vi "Convert to Lockin Data.vi"(7 "Raw data Y":i32[](array[numeric]), 8 "error in (no error)":errorcluster, 9 "Raw data X":i32[](array[numeric]), 10 "Raw data(F)":i32[](array[numeric]), 11 "RP Transceiver in":refnum<class "RP Transceiver.lvclass">) -> (0 "error out":errorcluster, 1 "Volatge X out":dbl[](array[numeric]), 2 "Frequency out":dbl[](array[numeric]), 3 "RP Transceiver out":refnum<class "RP Transceiver.lvclass">, 4 "Starting edges":i32[](array[numeric]), 5 "Ending edges":i32[](array[numeric]), 6 "Volatge Y out":dbl[](array[numeric]))   [LabVIEW 2024, in "RP Transceiver.lvclass"]
uses:
  RP Transceiver.lvclass
  RP Transceiver.lvclass/RP Transceiver.ctl
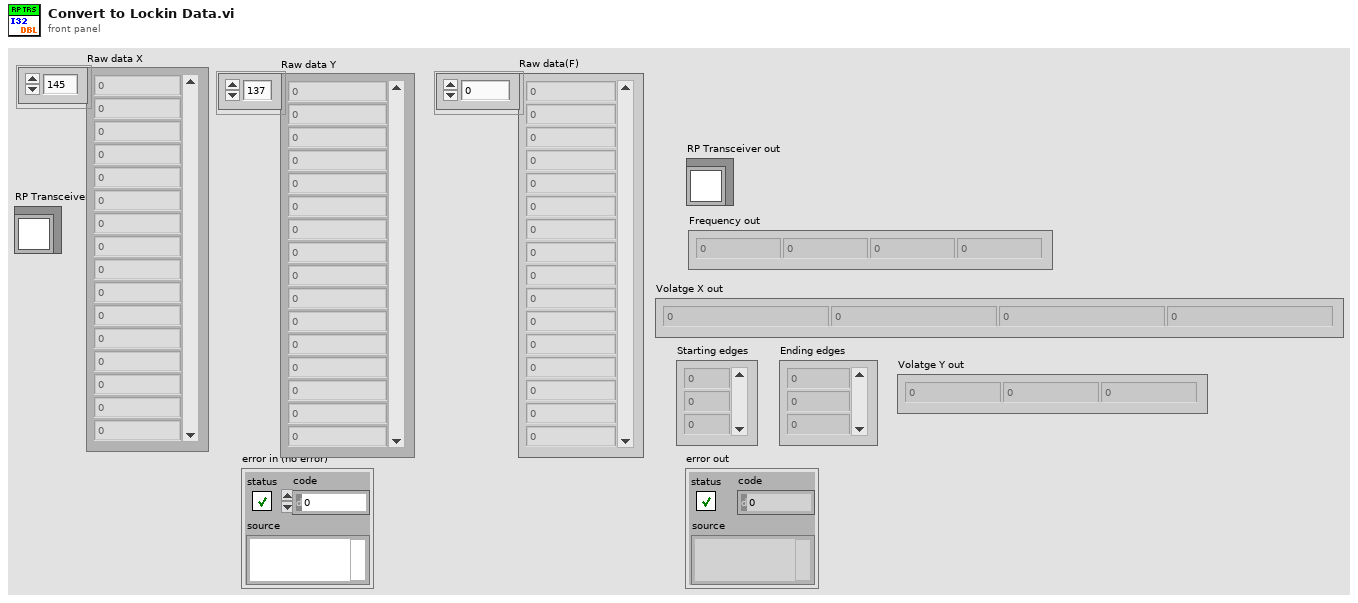
[diagram p1: front panel]
types:
  T1 = typedef "Receiver format.ctl" = enum16{"Hub port 2xy 4f", "Hub ports 234", "X-Y-F", "F-X-Y", "X-Y", "X"}
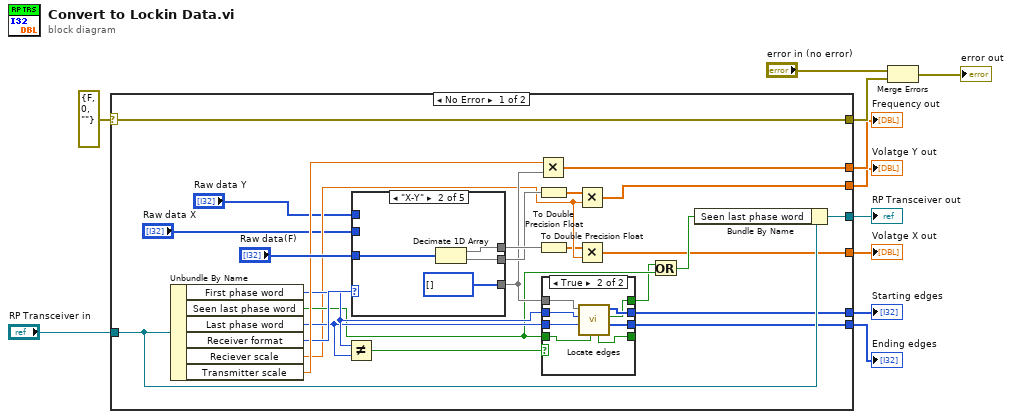
[diagram p0: block diagram]
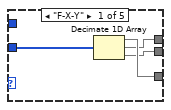
[diagram p3: hidden frame]
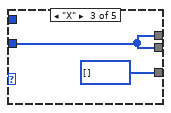
[diagram p4: hidden frame]
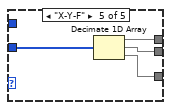
[diagram p6: hidden frame]
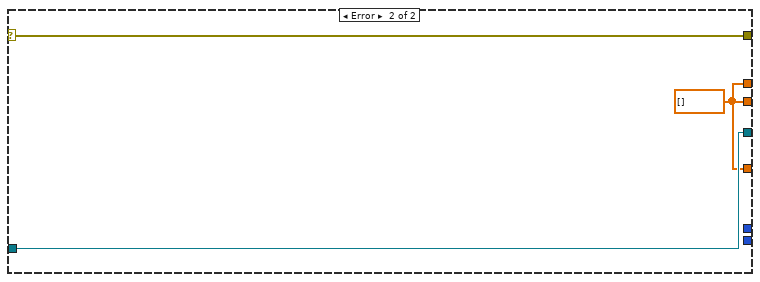
[diagram p7: hidden frame]
diagram:
  n1 = case shown="No Error" errorcluster {"status"=FALSE, "code"=0, "source"=""} ("error IO") {
    selector: errorcluster {"status"=FALSE, "code"=0, "source"=""} ("error IO") -> [w36 w65]
    tunnel: [w36 w65] -> w11
    tunnel: [w27 w64] -> w9
    tunnel: "RP Transceiver in" -> [w31 w64]
    tunnel: [w34 w63] -> w8
    tunnel: [w18 w63] -> w7
    tunnel: [w20 _] -> w6
    tunnel: [w19 _] -> w5
    tunnel: [w14 w63] -> w4
    frame No Error {
      n2 = Unbundle By Name(w31) -> ("First phase word"=w26:i32, "Seen last phase word"=w23:bool, "Last phase word"=w25:i32, "Receiver format"=w29:T1, "Reciever scale"=w16:dbl, "Transmitter scale"=w30:dbl)
      n3 = Not Equal?(x=w26, y=w25) -> (x != y?=w24:bool)
      n4 = case shown="\"X-Y\"" w29 {
        tunnel: "Raw data(F)" -> [w49 w53 w54 w58 w62]
        tunnel: [w48 i32[] [] i32[] [] w58 w61] -> w28
        tunnel: [w47 w52 w54 w56 w60] -> w33
        tunnel: [w46 w51 w54 w57 w59] -> w32
        tunnel: "Raw data Y" -> [_ _ _ w57 _]
        tunnel: "Raw data X" -> [_ _ _ w56 _]
        frame "F-X-Y" {
          n5 = Decimate 1D Array(w49) -> (w48:i32[], w47:i32[], w46:i32[])
        }
        frame "X-Y" {
          n6 = Decimate 1D Array(w53) -> (w52:i32[], w51:i32[])
        }
        frame "X" {
        }
        frame "Hub ports 234", Default {
        }
        frame "X-Y-F" {
          n7 = Decimate 1D Array(w62) -> (w60:i32[], w59:i32[], w61:i32[])
        }
      }
      n8 = Multiply(x=w30, y=w28) -> (x*y=w34:dbl[])
      n9 = To Double Precision Float(number=w32) -> (double precision float=w17:dbl[])
      n10 = To Double Precision Float(number=w33) -> (double precision float=w15:dbl[])
      n11 = case shown="True" w24 {
        tunnel: w28 -> [_ w45]
        tunnel: w26 -> [_ w44]
        tunnel: w25 -> [_ w43]
        tunnel: w23 -> [w37 w42]
        tunnel: [w37 w41] -> _
        tunnel: [_ w40] -> w20
        tunnel: [w37 w39] -> w21
        tunnel: [_ w38] -> w19
        frame False {
        }
        frame True {
          n12 = call "Locate edges.vi"("Seen last value"=w42, "Last value"=w43, "First value"=w44, "Values"=w45) -> ("Ending edges"=w38:i32[], "Seen last value 2"=w39:bool, "Starting edges"=w40:i32[], "Seen last value out"=w41:bool)  [unwired: 4 in]
        }
      }
      n13 = Multiply(x=w17, y=w16) -> (x*y=w14:dbl[])
      n14 = Multiply(x=w15, y=w16) -> (x*y=w18:dbl[])
      n15 = Or(x=w21, y=w23) -> (x .or. y?=w22:bool)
      n16 = Bundle By Name(cluster=w31, "Seen last phase word"=w22) -> (w27:refnum<class "RP Transceiver.lvclass">)
    }
    frame Error {
      w63 = dbl[] [] ("Data out")
    }
  }
  "RP Transceiver out" <- w9
  "Frequency out" <- w8
  "Volatge X out" <- w7
  "Ending edges" <- w5
  "Starting edges" <- w6
  "Volatge Y out" <- w4
  n17 = Merge Errors("error in (no error)", w11) -> (→"error out":errorcluster)
